vi "Write Panel Data.vi"(8 "Error In":errorcluster, 9 "Panel Data":variant, 10 "Field":string, 11 "Panel Helper in":refnum<class "Panel Helper.lvclass">) -> (0 "Error Out":errorcluster, 2 "Replaced?":bool)   [LabVIEW 2023, in "Panel Actor.lvlib" / "Panel.lvlib" / "Panel Helper.lvclass"]
doc: "Writes a field to the Panel Data.\n\n<B>Panel Helper In:</B> Panel Helper object to write panel data\n<B>Field:</B> Data field associated with the panel data.\n<B>Panel Data:</B> Panel data to write.\n<B>Error In:</B> Describes error conditions that occur before this node runs.\n\n<B>Replaced?:</B> Indicates if the Panel Data was replaced.\n<B>Error Out:</B> Contains error information.\n\n----\nPlease see the following web address for additional documentation and tutorial information:\nhttp://www.mooregoodideas.com/mgi-panel-manager/\n\nAuthor: Derek Trepanier\n\nCopyright (c) 2018, Moore Good Ideas, Inc.\n\nAll rights reserved.\n\nRedistribution and use in source and binary forms, with or without modification, are permitted provided that the following conditions are met:\n\n * Redistributions of source code must retain the above copyright notice, this list of conditions and the following disclaimer.\n * Redistributions in binary form must reproduce the above copyright notice, this list of conditions and the following disclaimer in the documentation and/or other materials provided with the distribution.\n * Neither the name of Moore Good Ideas, Inc. nor the names of its contributors may be used to endorse or promote products derived from this software without specific prior written permission.\n\nTHIS SOFTWARE IS PROVIDED BY THE COPYRIGHT HOLDERS AND CONTRIBUTORS \"AS IS\" AND ANY EXPRESS OR IMPLIED WARRANTIES, INCLUDING, BUT NOT LIMITED TO, THE IMPLIED WARRANTIES OF MERCHANTABILITY AND FITNESS FOR A PARTICULAR PURPOSE ARE DISCLAIMED. IN NO EVENT SHALL THE COPYRIGHT OWNER OR CONTRIBUTORS BE LIABLE FOR ANY DIRECT, INDIRECT, INCIDENTAL, SPECIAL, EXEMPLARY, OR CONSEQUENTIAL DAMAGES (INCLUDING, BUT NOT LIMITED TO, PROCUREMENT OF SUBSTITUTE GOODS OR SERVICES; LOSS OF USE, DATA, OR PROFITS; OR BUSINESS INTERRUPTION) HOWEVER CAUSED AND ON ANY THEORY OF LIABILITY, WHETHER IN CONTRACT, STRICT LIABILITY, OR TORT (INCLUDING NEGLIGENCE OR OTHERWISE) ARISING IN ANY WAY OUT OF THE USE OF THIS SOFTWARE, EVEN IF ADVISED OF THE POSSIBILITY OF SUCH DAMAGE."
uses:
  Panel Helper.lvclass
  Panel Helper.lvclass/Panel Helper.ctl
  Panel Updater/Panel Updater.lvclass
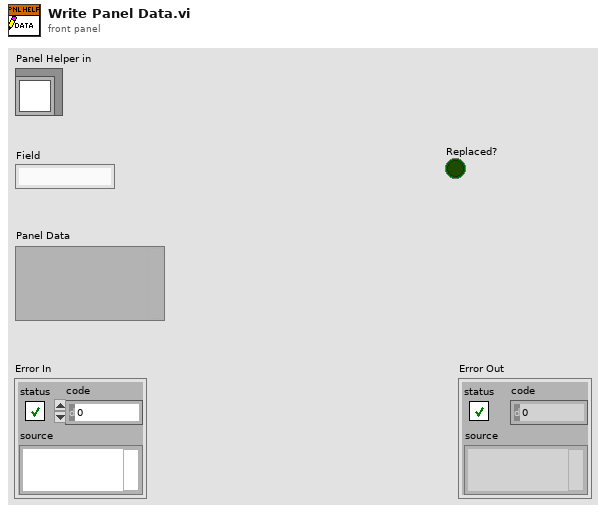
[diagram p1: front panel]
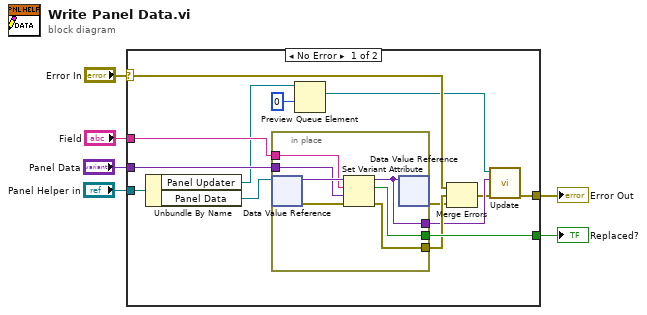
[diagram p0: block diagram]
diagram:
  n1 = case shown="No Error" "Error In" {
    selector: "Error In" -> [w20 w28]
    tunnel: [w12 w28] -> w3
    tunnel: "Panel Helper in" -> [w19 _]
    tunnel: "Field" -> [w17 _]
    tunnel: [w16 _] -> w2
    tunnel: "Panel Data" -> [w13 _]
    frame No Error {
      n2 = Unbundle By Name(w19) -> ("Panel Updater"=w8:refnum<queue>, "Panel Data"=w18:refnum<data-value>)
      n3 = in-place {
        in-place-border: w17 -> [w26]
        in-place-border: [w25] -> w16
        in-place-border: [w23] -> w15
        in-place-border: w13 -> [w22]
        in-place-border: [w21] -> w11
        n4 = in-place-dvr #1(w18) -> (w27:variant, w24:errorcluster)
        n5 = Set Variant Attribute(Variant=w27, name=w26, value=w22, error in=w24) -> (Variant out=w21:variant, replaced=w25:bool, error out=w23:errorcluster)
        n6 = in-place-dvr #1(w21) -> (w14:errorcluster)  [unwired: 1 out]
      }
      n7 = Preview Queue Element(queue=w8, timeout in ms (-1)=0) -> (element=w7:refnum<class "Panel Updater.lvclass">)  [unwired: 1 in, 3 out]
      n8 = Merge Errors(w20, w15, w14) -> (w10:errorcluster)
      n9 = call-dynamic "Update.vi"("error in (no error)"=w10, "Panel Data"=w11, "Panel Updater in"=w7) -> ("error out"=w12:errorcluster)  [unwired: 8 in]
    }
    frame Error {
    }
  }
  "Error Out" <- w3
  "Replaced?" <- w2
